vi "TEST - Array of VData to VArray.vi"(8 "error in (no error)":errorcluster) -> (0 "error out":errorcluster, 2 "pass":bool)   [LabVIEW 2020, in "test_openg_variant.lvlib"]
uses:
  test_openg_variant.lvlib
  <vilib>/addons/_JKI Toolkits/Caraya/classes/Assert/Assert True.vi
  source/library/openg_variant.lvlib
  <vilib>/addons/_JKI Toolkits/Caraya/classes/Test/Test.lvclass
  <vilib>/addons/_JKI Toolkits/Caraya/classes/Assert/Assert.lvclass
panel:
  out "expected result":errorcluster[](array[cluster])
  out "result":errorcluster[](array[cluster])
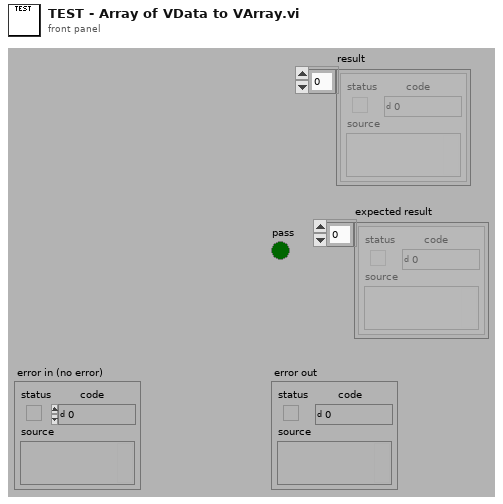
[diagram p1: front panel]
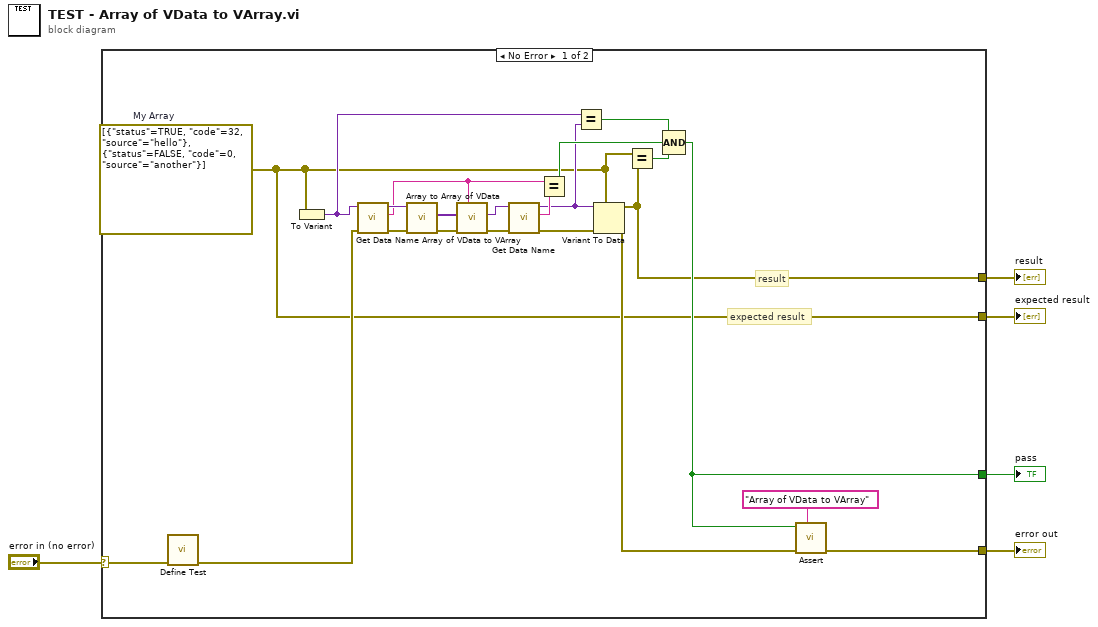
[diagram p0: block diagram]
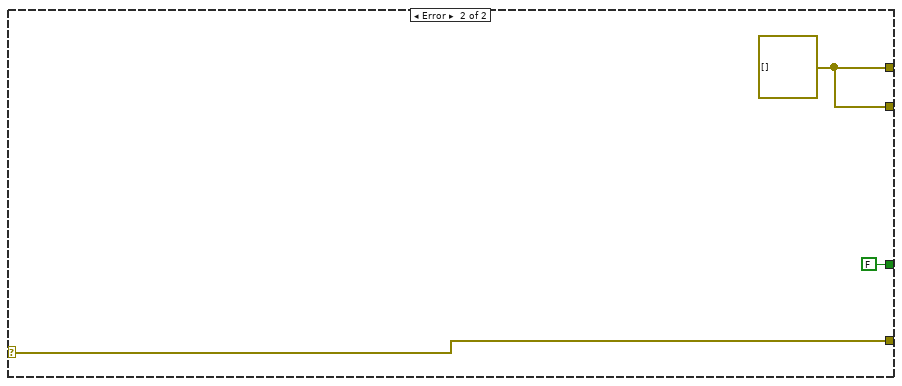
[diagram p2: hidden frame]
diagram:
  n1 = case shown="No Error" "error in (no error)" {
    selector: "error in (no error)" -> [w12 w30]
    tunnel: [w8 FALSE] -> w5
    tunnel: [w10 w30] -> w3
    tunnel: [w6 w28] -> w1
    tunnel: [w7 w28] -> w2
    frame No Error {
      w7 = errorcluster[] [{"status"=TRUE, "code"=32, "source"="hello"}, {"status"=FALSE, "code"=0, "source"="another"}]  # My Array
      # "result"
      # "expected result"
      n2 = call <vilib>:"Define Test.vi"("error in (no error)"=w12) -> ("error out"=w11:errorcluster)  [unwired: 9 in, 1 out]
      n3 = To Variant(anything=w7) -> (Variant=w22:variant)
      n4 = call "Get Data Name.vi"("error in (no error)"=w11, "Data"=w22) -> ("error out"=w21:errorcluster, "Data Name"=w16:string, "Data dup"=w23:variant)  [unwired: 7 in]
      n5 = call "Array to Array of VData.vi"("error in (no error)"=w21, "MultiD Array"=w23) -> ("error out"=w24:errorcluster, "1D Array of Variants"=w25:variant[])  [unwired: 8 in]
      n6 = call "Array of VData to VArray.vi"("Array Name"=w16, "error in (no error)"=w24, "1D Array of VData"=w25) -> ("error out"=w19:errorcluster, "VArray"=w20:variant)  [unwired: 7 in]
      n7 = call "Get Data Name.vi"("error in (no error)"=w19, "Data"=w20) -> ("error out"=w18:errorcluster, "Data Name"=w17:string, "Data dup"=w14:variant)  [unwired: 7 in]
      n8 = Equal?(x=w16, y=w17) -> (x = y?=w15:bool)
      n9 = Equal?(x=w22, y=w14) -> (x = y?=w26:bool)
      n10 = Variant To Data(error in=w18, type=w7, Variant=w14) -> (data=w6:errorcluster[], error out=w9:errorcluster)
      n11 = Equal?(x=w7, y=w6) -> (x = y?=w27:bool)
      n12 = Compound Arithmetic op=AND(w26, w15, w27) -> (w8:bool)
      n13 = call-poly <vilib>:"Assert.vi"("Label"="Array of VData to VArray" ("Label (VI Title)"), "error in (no error)"=w9, "True?"=w8) -> ("error out"=w10:errorcluster)  [unwired: 7 in, 1 out]
    }
    frame Error {
      w28 = errorcluster[] [] ("My Array")
    }
  }
  "pass" <- w5
  "error out" <- w3
  "expected result" <- w2
  "result" <- w1
